vi "startS1010.vi"(8 "error in (no error)":errorcluster, 11 "AtomChipHWC in":refnum<class "AtomChipHWC.lvclass">) -> (0 "error out":errorcluster, 3 "AtomChipHWC out":refnum<class "AtomChipHWC.lvclass">)   [LabVIEW 2009, in "Hardware.lvlib" / "HWControllers.lvlib" / "AtomChipHWC.lvclass"]
doc: "Start sound card"
uses:
  AtomChipHWC.lvclass
  AtomChipHWC.lvclass/AtomChipHWC.ctl
  Channels/VoltOutput/AnalogOutput.lvclass
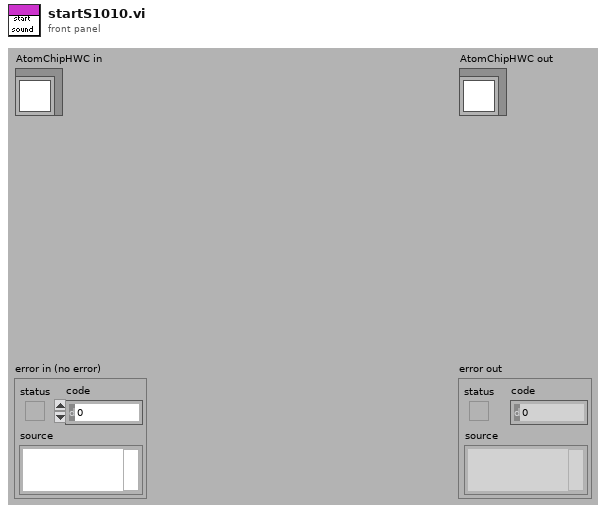
[diagram p1: front panel]
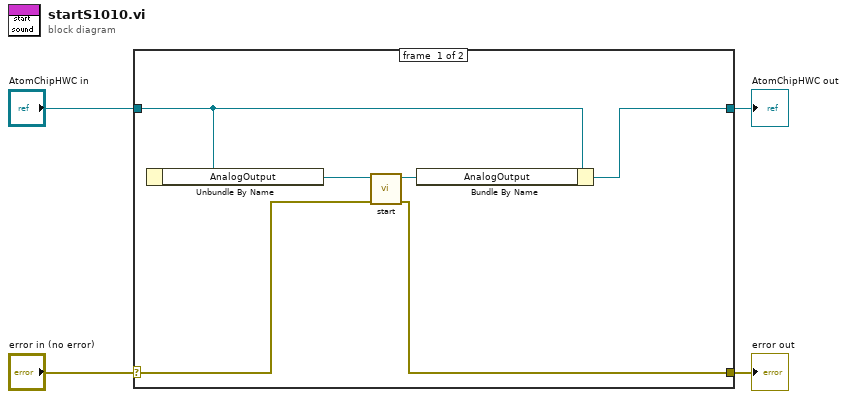
[diagram p0: block diagram]
diagram:
  n1 = case shown="No Error" "error in (no error)" {
    selector: "error in (no error)" -> [w9 w12]
    tunnel: [w8 w12] -> w3
    tunnel: [w5 w11] -> w1
    tunnel: "AtomChipHWC in" -> [w6 w11]
    frame #0 {
      n2 = Unbundle By Name(w6) -> ("AnalogOutput"=w10:refnum<class "AnalogOutput.lvclass">)
      n3 = call-dynamic "start.vi"("error in (no error)"=w9, "AnalogOutput in"=w10) -> ("error out"=w8:errorcluster, "AnalogOutput out"=w7:refnum<class "AnalogOutput.lvclass">)  [unwired: 8 in]
      n4 = Bundle By Name(cluster=w6, "AnalogOutput"=w7) -> (w5:refnum<class "AtomChipHWC.lvclass">)
    }
    frame #1 {
    }
  }
  "error out" <- w3
  "AtomChipHWC out" <- w1
